vi "Correct Data process.vi"(8 "error in":errorcluster, 11 "区域选择":enum16{"1st", "2nd"}(ring)) -> (0 "error out":errorcluster)   [LabVIEW 2015, in "Debug.lvlib"]
uses:
  Debug.lvlib
  Support/Correct Data Process State.ctl
  <vilib>/Analysis/1siggen.llb/Ramp Pattern by Samples.vi
  <vilib>/Utility/file.llb/Read Delimited Spreadsheet (DBL).vi
  <vilib>/gmath/NI_Gmath.lvlib
  <vilib>/Analysis/NI_AALBase.lvlib
  Sub VIs/Boimetry Processing/Boimetry Processing.lvlib
panel:
  in  "停止按钮":bool
  in  "计算":bool
  in  "结束位置":i32
  in  "开始位置":i32
  in  "单位长度":dbl=0.01 format="%#_13g"
  out "分析图 2":dbl[](graph)
  out "分析图":dbl[][](graph)
  # "Ascan Correct Process"
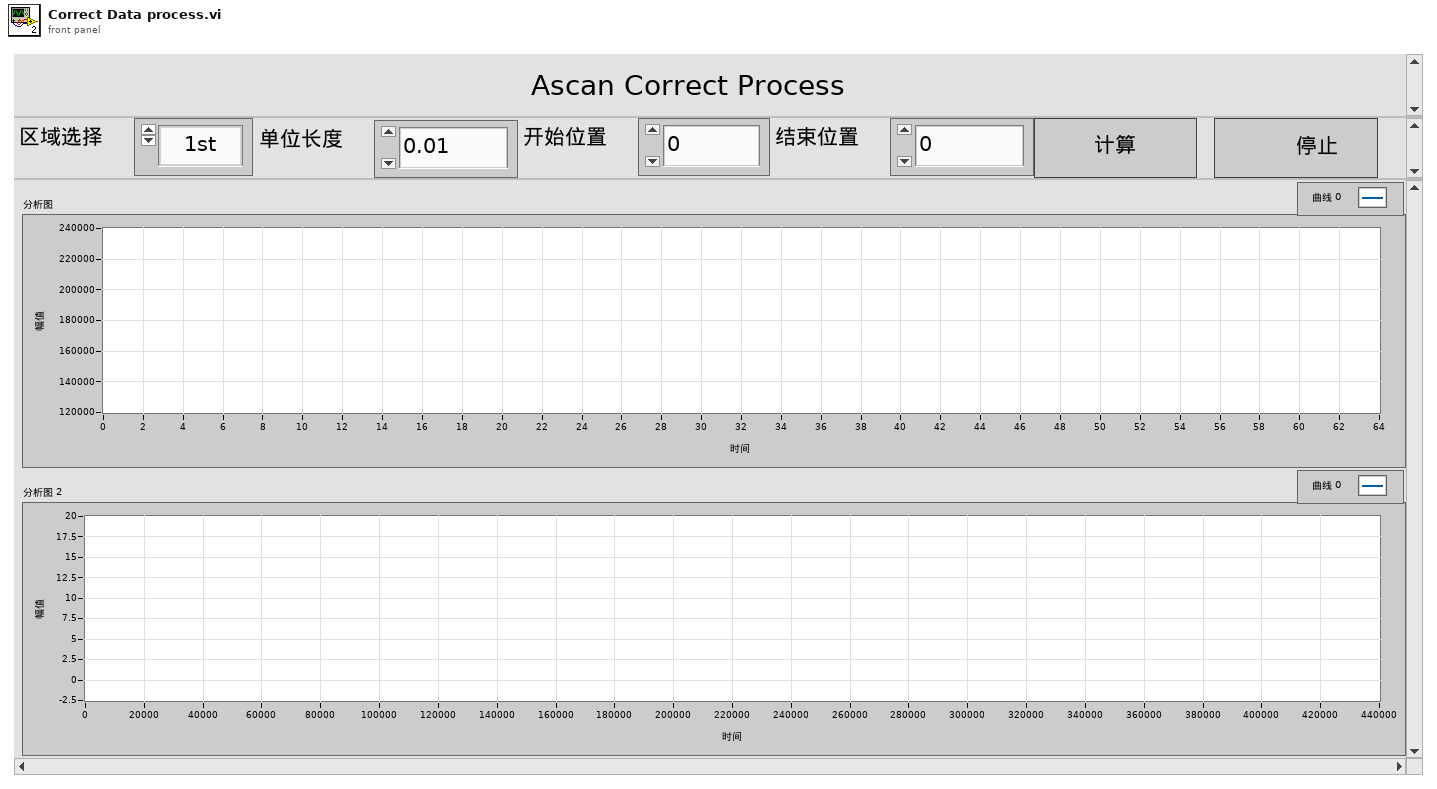
[diagram p1: front panel]
types:
  T1 = typedef "Debug.lvlib/Correct Data Process State.ctl" = enum16{"Initialize", "Update Settings", "Calculate", "Load Data", "Wait For Event", "Exit"}
  T2 = typedef "Boimetry Processing.lvlib/Biometry Configuration.ctl" = cluster{"Interference Width":i32, "Interference Threshold":dbl, "Cornea Len Division":i32, "Correction Data 1st Path":string, "1st_Start_Position":dbl, "Correction Data 2nd Path":string, "2nd_Start_Position":dbl, "Index Corneal":dbl, "Index Water":dbl, "Index Len":dbl, "Working Position":cluster{"FirstStart":i32, "FirstEnd":i32, "SecondStart":i32, "SecondEnd":i32}}
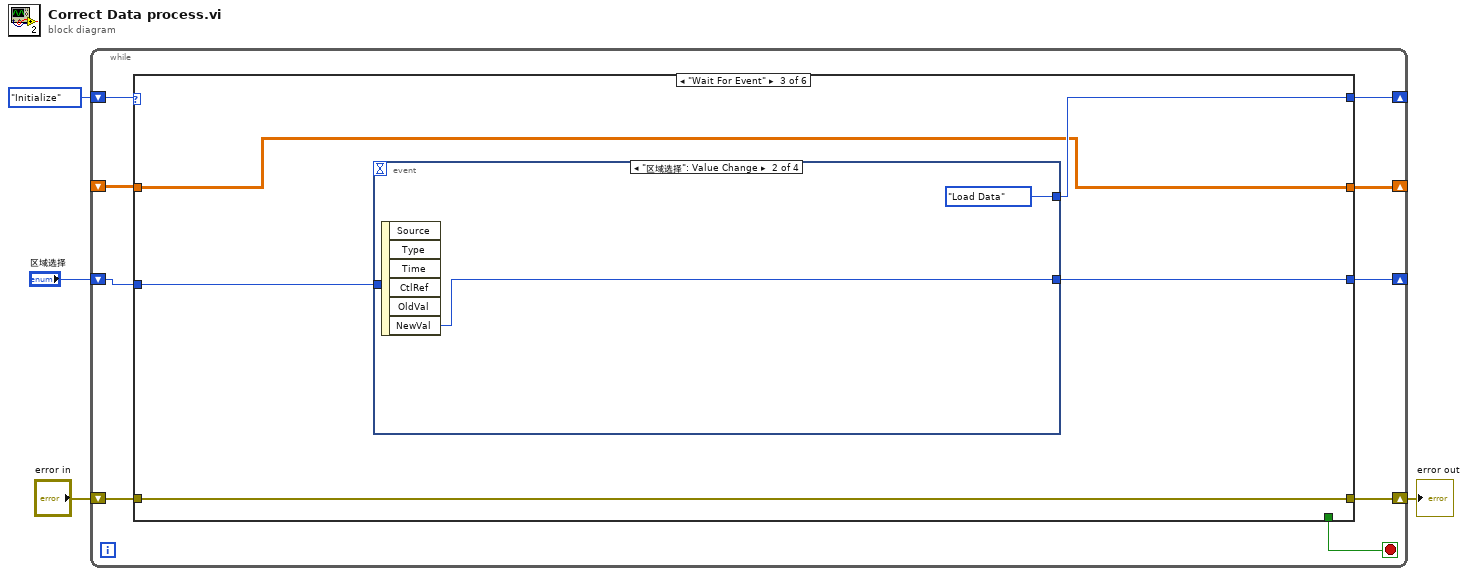
[diagram p0: block diagram]
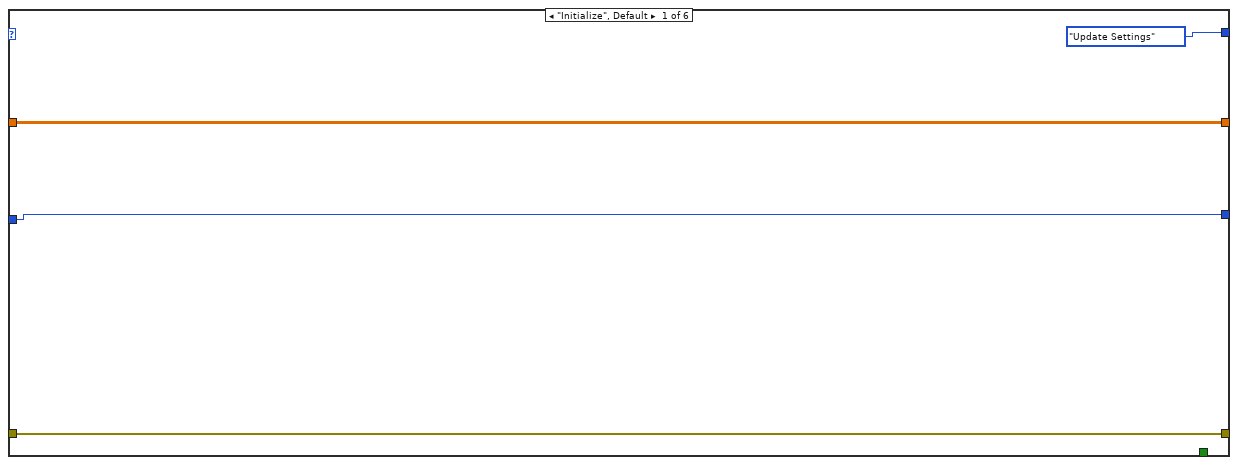
[diagram p2: hidden frame]
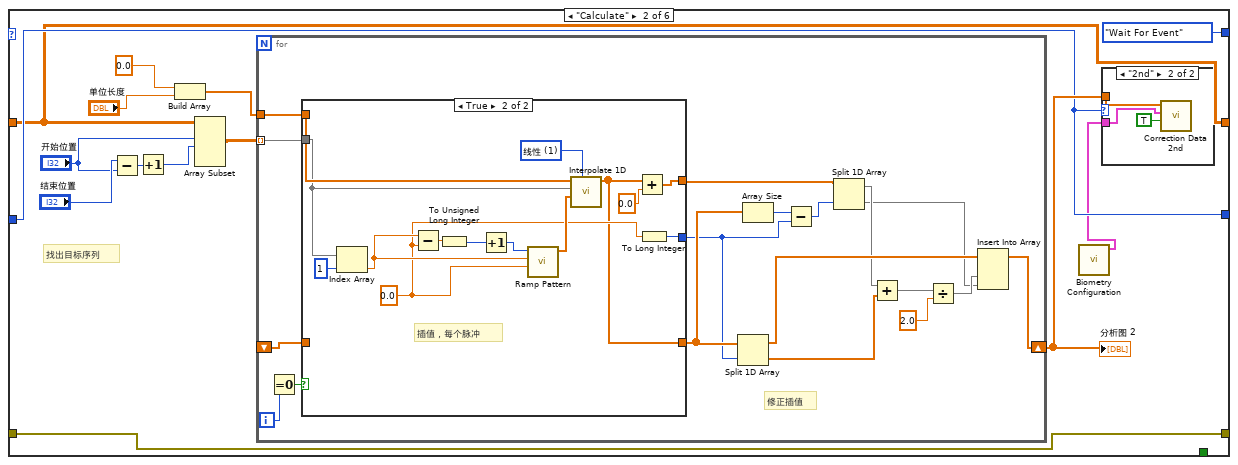
[diagram p3: hidden frame]
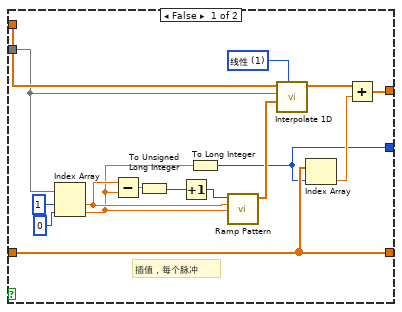
[diagram p4: hidden frame]
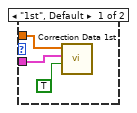
[diagram p5: hidden frame]
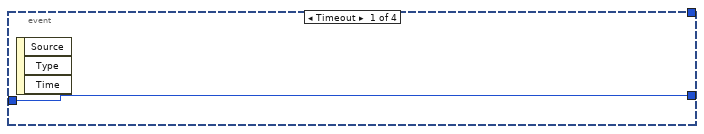
[diagram p6: hidden frame]
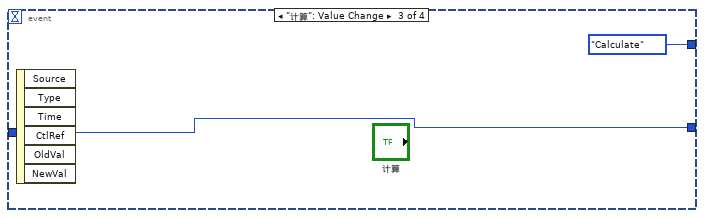
[diagram p7: hidden frame]
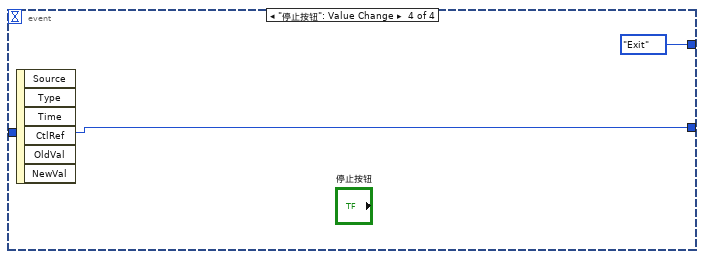
[diagram p8: hidden frame]
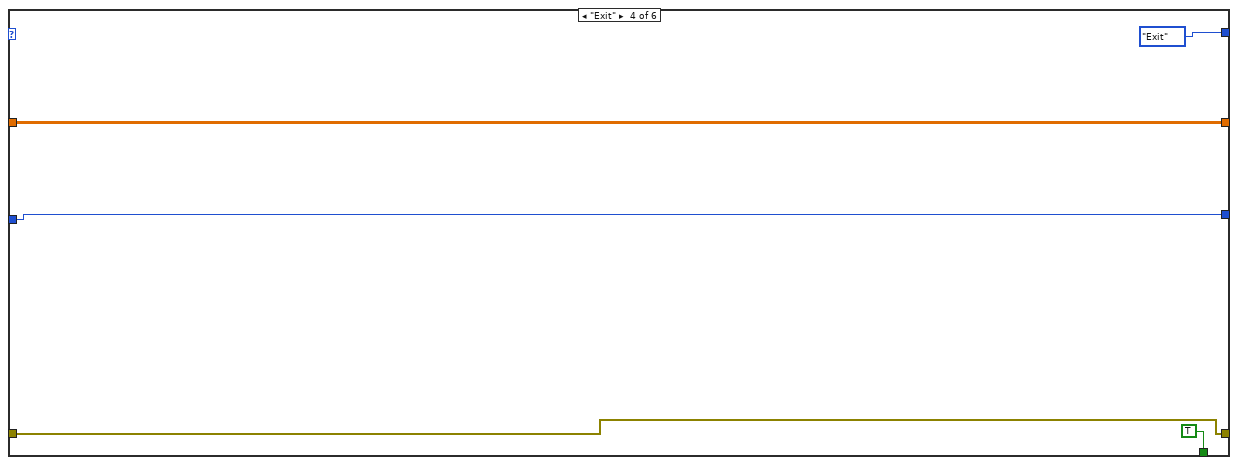
[diagram p9: hidden frame]
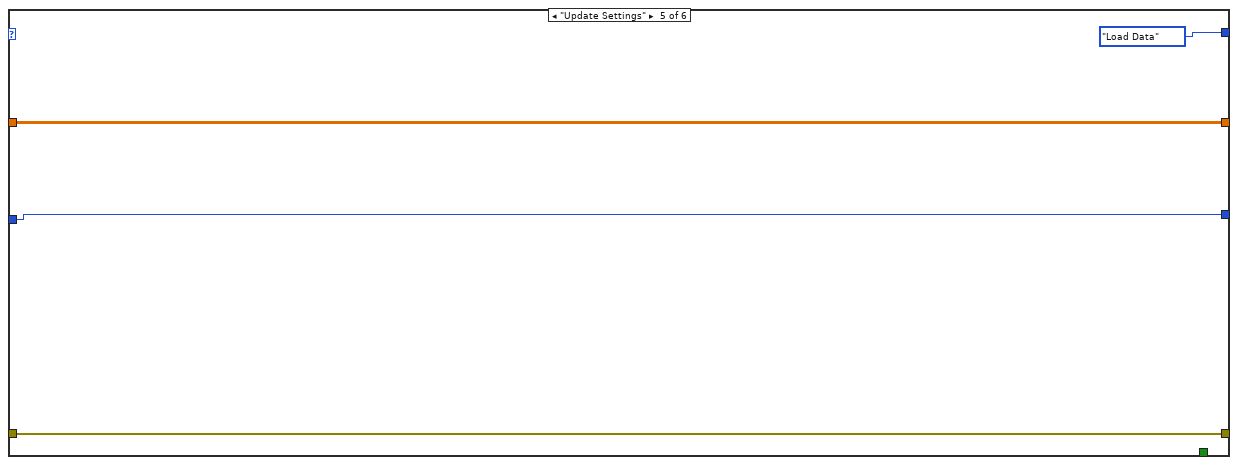
[diagram p10: hidden frame]
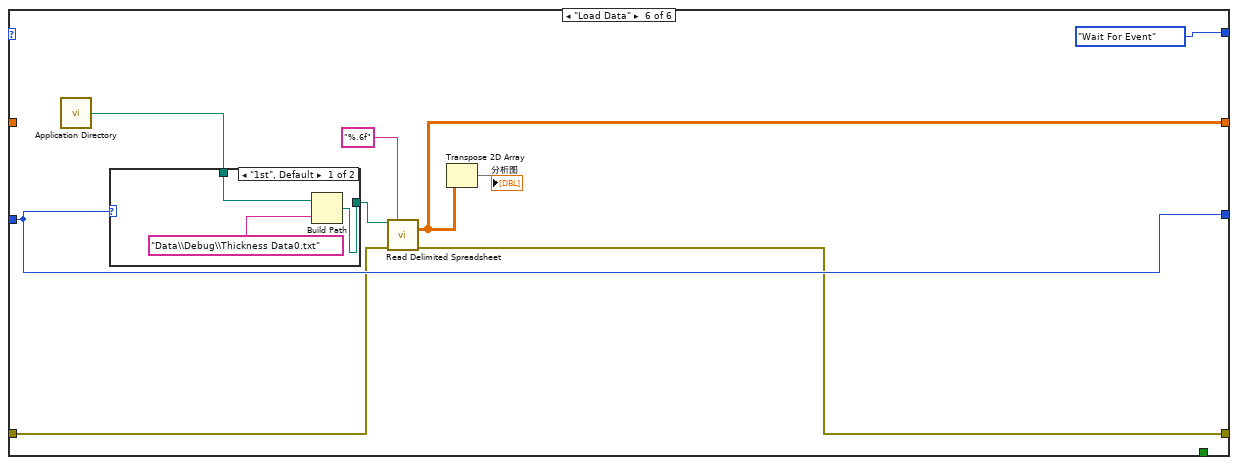
[diagram p11: hidden frame]
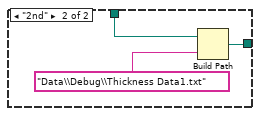
[diagram p12: hidden frame]
diagram:
  n1 = while {
    shift-right: [w10] -> _
    shift-left: _ -> [w13]
    shift-right: [w11] -> _
    shift-left: Correct_Data_Process_State."Initialize" ("Calculation Distance State") -> [w12]
    shift-right: [w9] -> _
    shift-left: "区域选择" -> [w8]
    shift-right: [w6] -> w2
    shift-left: "error in" -> [w5]
    stop <- w7 stop-if-true
    n2 = case shown="\"Wait For Event\"" w12 {
      tunnel: w13 -> [w15 w20 w87 w101 w105 _]
      tunnel: [Correct_Data_Process_State."Update Settings" ("Calculation Distance State") Correct_Data_Process_State."Wait For Event" ("Calculation Distance State") w88 Correct_Data_Process_State."Exit" ("Calculation Distance State") Correct_Data_Process_State."Load Data" ("Calculation Distance State") Correct_Data_Process_State."Wait For Event" ("Calculation Distance State")] -> w11
      tunnel: [w15 w20 w87 w101 w105 w111] -> w10
      tunnel: [w16 w21 w90 w100 w104 w110] -> w9
      tunnel: w8 -> [w16 w21 w89 w100 w104 w110]
      tunnel: [_ _ _ TRUE _ _] -> w7
      tunnel: [w14 w18 w86 w98 w103 w108] -> w6
      tunnel: w5 -> [w14 w18 w86 w98 w103 w107]
      frame "Initialize", Default {
      }
      frame "Calculate" {
        # "找出目标序列"
        n3 = Subtract(x="结束位置", y="开始位置") -> (x-y=w30:i32)
        n4 = Increment(x=w30) -> (x+1=w26:i32)
        n5 = Build Array(0.0 ("元素"), "单位长度") -> (w27:dbl[])
        n6 = Array Subset(array=w20, index (row)="开始位置", length (row)=w26) -> (w24:dbl[][])  [unwired: 2 in]
        n7 = for {
          tunnel: w24 -> [w47] mode=indexing
          tunnel: w27 -> [w46]
          shift-right: [w38] -> w23
          shift-left: _ -> [w45]
          i -> [w49]
          # "修正插值"
          n8 = Equal To 0?(x=w49) -> (x = 0?=w48:bool)
          n9 = case shown="True" w48 {
            tunnel: w47 -> [w62 w76]
            tunnel: w46 -> [w65 w79]
            tunnel: [w55 w66] -> w32
            tunnel: [w52 w67] -> w41
            tunnel: w45 -> [w52 _]
            tunnel: [w50 w70] -> w33
            frame False {
              w58 = 1 items=["最近", "线性", "样条", "cubic Hermite", "拉格朗日"] ("method")
              # "插值，每个脉冲"
              n10 = Index Array(array=w62, index #1=1 ("索引"), index #2=0 ("索引")) -> (element #1=w56:dbl, element #2=w53:dbl)
              n11 = Subtract(x=w56, y=w53) -> (x-y=w60:dbl)
              n12 = To Unsigned Long Integer(number=w60) -> (unsigned 32bit integer=w63:u32)
              n13 = Increment(x=w63) -> (x+1=w64:u32)
              n14 = To Long Integer(number=w53) -> (32bit integer=w50:i32)
              n15 = call-poly <vilib>:"Ramp Pattern.vi"("start"=w53, "end"=w56, "samples"=w64) -> ("Ramp Pattern"=w59:dbl[])  [unwired: 7 in, 1 out]
              n16 = call <vilib>:"Interpolate 1D.vi"("method"=w58, "xi"=w59, "X"=w62, "Y"=w65) -> ("yi"=w54:dbl[])  [unwired: 5 in, 2 out]
              n17 = Index Array(array=w52, index=w50) -> (element=w51:dbl)
              n18 = Add(x=w54, y=w51) -> (x+y=w55:dbl[])
            }
            frame True {
              w69 = 0.0 ("start")
              w72 = 1 items=["最近", "线性", "样条", "cubic Hermite", "拉格朗日"] ("method")
              # "插值，每个脉冲"
              n19 = Index Array(array=w76, index=1 ("索引")) -> (element=w71:dbl)
              n20 = Subtract(x=w71, y=w69) -> (x-y=w74:dbl)
              n21 = To Unsigned Long Integer(number=w74) -> (unsigned 32bit integer=w77:u32)
              n22 = Increment(x=w77) -> (x+1=w78:u32)
              n23 = call-poly <vilib>:"Ramp Pattern.vi"("start"=w69, "end"=w71, "samples"=w78) -> ("Ramp Pattern"=w73:dbl[])  [unwired: 7 in, 1 out]
              n24 = call <vilib>:"Interpolate 1D.vi"("method"=w72, "xi"=w73, "X"=w76, "Y"=w79) -> ("yi"=w67:dbl[])  [unwired: 5 in, 2 out]
              n25 = Add(x=w67, y=0.0) -> (x+y=w66:dbl[])
              n26 = To Long Integer(number=w69) -> (32bit integer=w70:i32)
            }
          }
          n27 = Split 1D Array(array=w41, index=w33) -> (first subarray=w40:dbl[], second subarray=w42:dbl[])
          n28 = Array Size(array=w41) -> (size(s)=w37:i32)
          n29 = Subtract(x=w37, y=w33) -> (x-y=w36:i32)
          n30 = Split 1D Array(array=w32, index=w36) -> (first subarray=w35:dbl[], second subarray=w34:dbl[])
          n31 = Add(x=w35, y=w42) -> (x+y=w44:dbl[])
          n32 = Divide(x=w44, y=2.0) -> (x/y=w39:dbl[])
          n33 = Insert Into Array(array=w40, new element #1=w39, new element #2=w34) -> (w38:dbl[])  [unwired: 1 in]
        }
        "分析图 2" <- w23
        n34 = call "Biometry Configuration.vi"() -> ("Biometry Configuration"=w19:T2)  [unwired: 10 in, 1 out]
        n35 = case shown="\"2nd\"" w21 {
          tunnel: w23 -> [w82 w85]
          tunnel: w19 -> [w80 w83]
          frame "1st", Default {
            n36 = call "Correction Data 1st.vi"("写入（非为读取）"=TRUE, "Biometry Configuration"=w80, "Input Correction Data"=w82) -> ()  [unwired: 7 in, 2 out]
          }
          frame "2nd" {
            n37 = call "Correction Data 2nd.vi"("写入（非为读取）"=TRUE, "Biometry Configuration"=w83, "Input Correction Data"=w85) -> ()  [unwired: 7 in, 2 out]
          }
        }
      }
      frame "Wait For Event" {
        n38 = event shown="[1] \"区域选择\": Value Change" {
          selector: _ -> [_ _ _ _]
          dyn-events: _ -> [_ _ _ _]
          timeout: _ -> [_ _ _ _]
          tunnel: [w91 w92 w94 w96] -> w90
          tunnel: w89 -> [w91 _ w94 w96]
          tunnel: [_ Correct_Data_Process_State."Load Data" ("Calculation Distance State") Correct_Data_Process_State."Calculate" ("Calculation Distance State") Correct_Data_Process_State."Exit" ("Calculation Distance State")] -> w88
          event Timeout {
            n39 = event-data() -> ()  [unwired: 1 in, 3 out]
          }
          event "区域选择": Value Change {
            n40 = event-data() -> ("NewVal"=w92:enum16{"1st", "2nd"})  [unwired: 1 in, 5 out]
          }
          event "计算": Value Change {
            n41 = event-data() -> ()  [unwired: 1 in, 6 out]
          }
          event "停止按钮": Value Change {
            n42 = event-data() -> ()  [unwired: 1 in, 6 out]
          }
        }
      }
      frame "Exit" {
      }
      frame "Update Settings" {
      }
      frame "Load Data" {
        n43 = call <vilib>:"Application Directory.vi"() -> ("Application Directory"=w113:path)
        n44 = case shown="\"1st\", Default" w110 {
          tunnel: w113 -> [w118 w120]
          tunnel: [w116 w119] -> w114
          frame "1st", Default {
            n45 = Build Path(base path=w118, name or relative path="Data\\Debug\\Thickness Data0.txt" ("名称或相对路径")) -> (appended path=w116:path)
          }
          frame "2nd" {
            n46 = Build Path(base path=w120, name or relative path="Data\\Debug\\Thickness Data1.txt" ("名称或相对路径")) -> (appended path=w119:path)
          }
        }
        n47 = call-poly <vilib>:"Read Delimited Spreadsheet.vi"("file path (dialog if empty)"=w114, "format (%.3f)"="%.6f", "error in (no error)"=w107) -> ("all rows"=w111:dbl[][], "error out"=w108:errorcluster)  [unwired: 7 in, 4 out]
        n48 = Transpose 2D Array(2D array=w111) -> (transposed array=→"分析图":dbl[][])
      }
    }
  }
  "error out" <- w2
